vi "Change Parent.vi"(8 "error in (no error)":errorcluster, 9 "New Parent":refnum<data-value>, 10 "Node":refnum<data-value>, 11 "AST in":refnum<class "AST.lvclass">) -> (0 "error out":errorcluster, 3 "AST out":refnum<class "AST.lvclass">)   [LabVIEW 2020, in "PicoG-ParserLexer.lvlib" / "AST.lvclass"]
uses:
  AST.lvclass
  Node/Node.lvclass
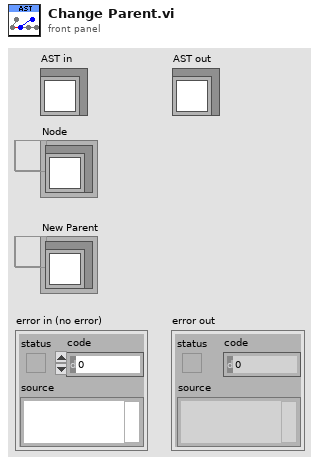
[diagram p1: front panel]
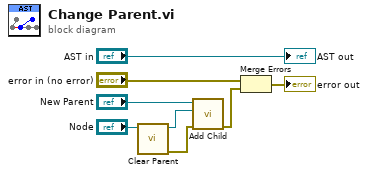
[diagram p0: block diagram]
diagram:
  n1 = call "Clear Parent.vi"("NodeRef In"="Node") -> ("error out"=w2:errorcluster, "NodeRef"=w4:refnum<data-value>)  [unwired: 9 in]
  n2 = call "Add Child.vi"("error in (no error)"=w2, "Child"=w4, "NodeRef In"="New Parent") -> ("error out"=w1:errorcluster)  [unwired: 7 in, 1 out]
  n3 = Merge Errors("error in (no error)", w1) -> (→"error out":errorcluster)
  "AST out" <- "AST in"
